vi "Get This Application.vi"(11 "jettl in":refnum<class "jettl.lvclass">) -> (2 "This Application":refnum<vi>)   [LabVIEW 2021, in "jettl.lvlib" / "jettl.lvclass"]
uses:
  jettl.lvclass
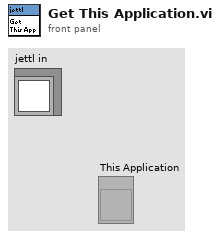
[diagram p1: front panel]
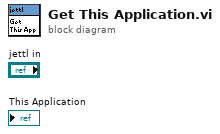
[diagram p0: block diagram]
diagram:
